vi "Bitfiles Paths.vi"(8 "select bitfile":u8) -> (0 "Bitfile path":path)   [LabVIEW 2015]
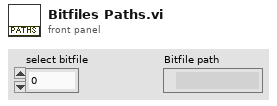
[diagram p1: front panel]
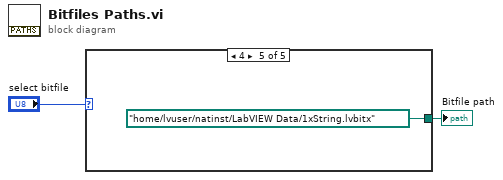
[diagram p0: block diagram]
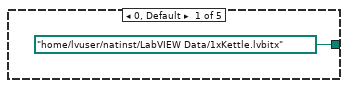
[diagram p2: hidden frame]
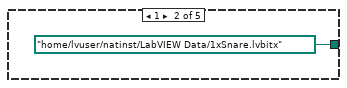
[diagram p3: hidden frame]
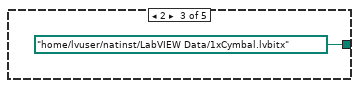
[diagram p4: hidden frame]
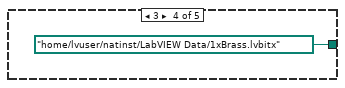
[diagram p5: hidden frame]
diagram:
  n1 = case shown="4" "select bitfile" {
    tunnel: [path "/home/lvuser/natinst/LabVIEW Data/1xKettle.lvbitx" ("Bitfile path") path "/home/lvuser/natinst/LabVIEW Data/1xSnare.lvbitx" ("Bitfile path") path "/home/lvuser/natinst/LabVIEW Data/1xCymbal.lvbitx" ("Bitfile path") path "/home/lvuser/natinst/LabVIEW Data/1xBrass.lvbitx" ("Bitfile path") path "/home/lvuser/natinst/LabVIEW Data/1xString.lvbitx" ("Bitfile path")] -> w1
    frame 0, Default {
    }
    frame 1 {
    }
    frame 2 {
    }
    frame 3 {
    }
    frame 4 {
    }
  }
  "Bitfile path" <- w1
